vi "Create Robot State Machine.vi"(8 "error in (no error)":errorcluster, 11 "Robot Definition":T1) -> (0 "error out":errorcluster, 3 "Cluster":T2)   [LabVIEW 2014]
uses:
  Robot_creation_loop_data.ctl
  Robot_definition.ctl
  Build robot states.ctl
  <vilib>/picture/3D Picture Control/Object/Create Object (name).vi
  <vilib>/picture/3D Picture Control/Object/Add Object (no reference).vi
  <vilib>/picture/3D Picture Control/Object/Create Object (drawable).vi
  <vilib>/picture/3D Picture Control/Object/Add Object (reference).vi
  <vilib>/picture/3D Picture Control/NI_3D Picture Control.lvlib
panel:
  out "x/y":sgl
  out "Robot Definition.Base":sgl
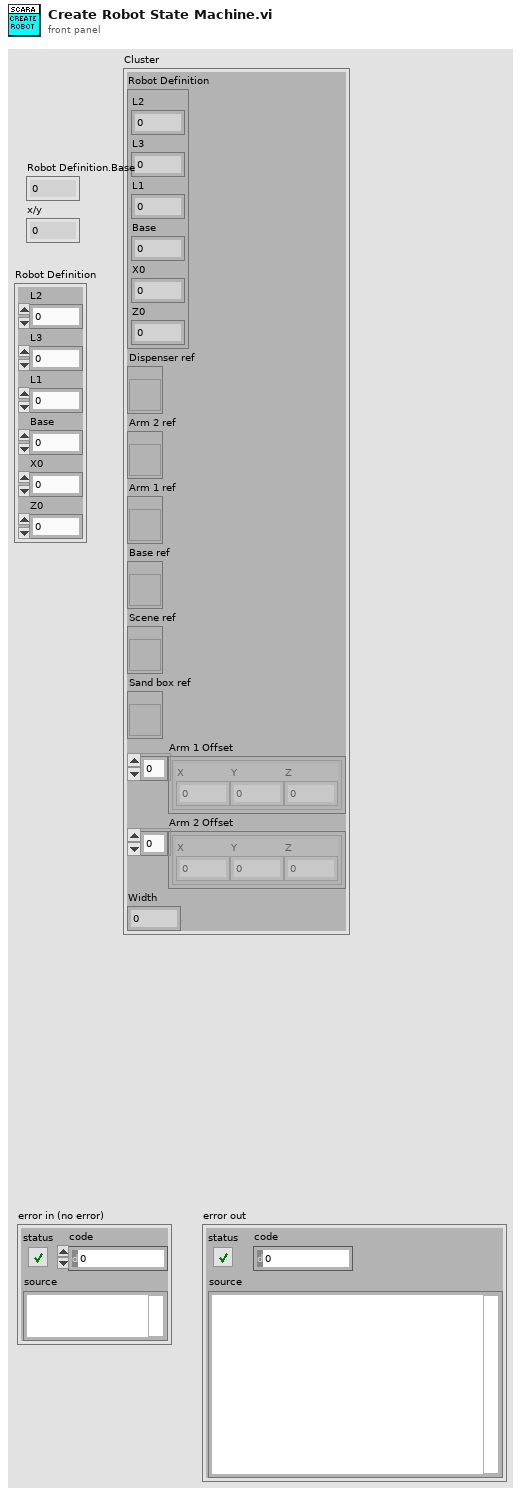
[diagram p1: front panel]
types:
  T1 = typedef "Robot_definition.ctl" = cluster{"L2":sgl, "L3":sgl, "L1":sgl, "Base":sgl, "X0":sgl, "Z0":sgl}
  T2 = typedef "Robot_creation_loop_data.ctl" = cluster{"Robot Definition":T1, "Dispenser ref":refnum<vi>, "Arm 2 ref":refnum<vi>, "Arm 1 ref":refnum<vi>, "Base ref":refnum<vi>, "Scene ref":refnum<vi>, "Sand box ref":refnum<vi>, "Arm 1 Offset":cluster{"X":sgl, "Y":sgl, "Z":sgl}[], "Arm 2 Offset":cluster{"X":sgl, "Y":sgl, "Z":sgl}[], "Width":sgl}
  T3 = typedef "Build robot states.ctl" = enum16{"Init 1 - Clear references", "Create Scene", "Create Sand box", "Create Base", "Create Arm 1", "Create Arm 2", "Create Dispenser", "Exit"}
  T4 = cluster{"Red":sgl, "Green":sgl, "Blue":sgl, "Alpha":sgl}
  T5 = enum16{"Zero", "One", "Destination Color", "One Minus Destination Color", "Source Alpha", "One Minus Source Alpha", "Destination Alpha", "One Minus Destination Alpha", "Source Alpha Saturate"}
  T6 = enum16{"Zero", "One", "Source Color", "One Minus Source Color", "Source Alpha", "One Minus Source Alpha", "Destination Alpha", "One Minus Destination Alpha"}
  T7 = enum16{"Normal Bin", "Opaque Bin", "Transparent Bin"}
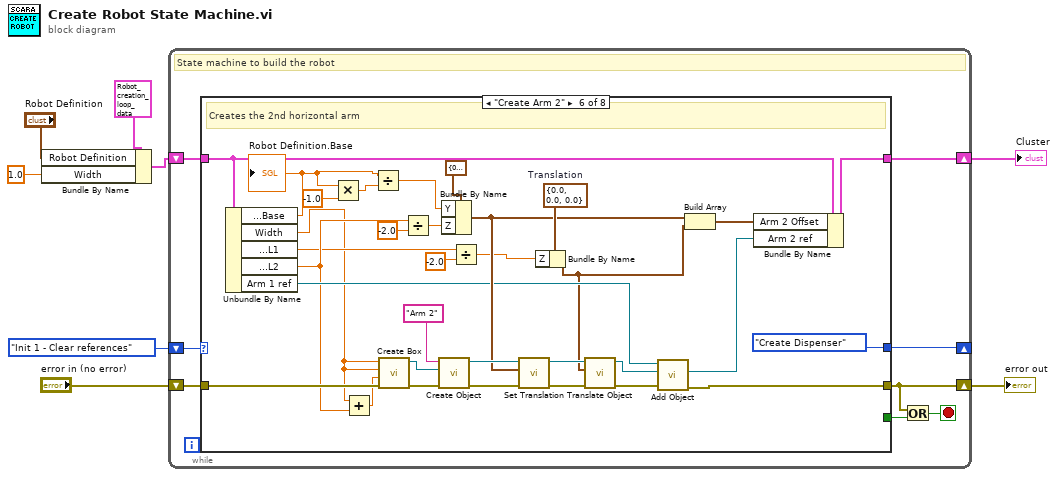
[diagram p0: block diagram]
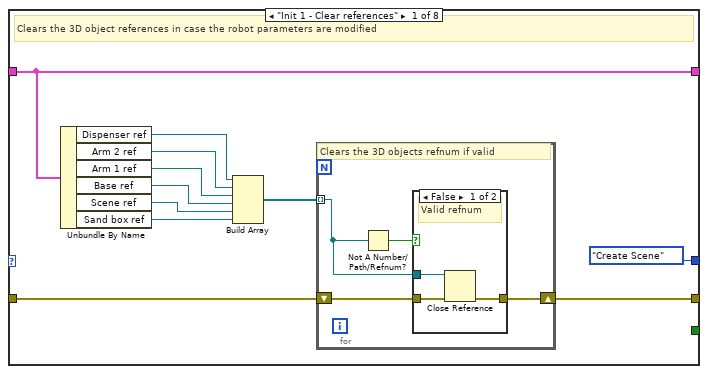
[diagram p2: hidden frame]
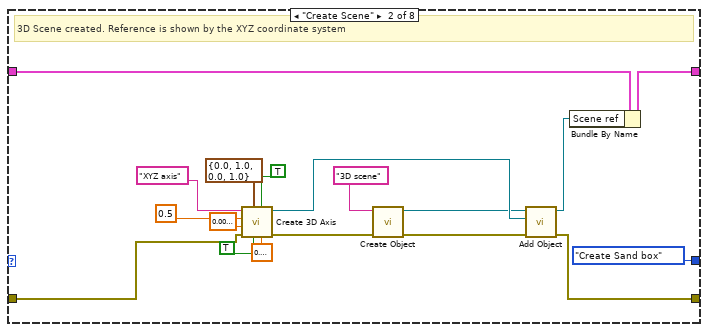
[diagram p4: hidden frame]
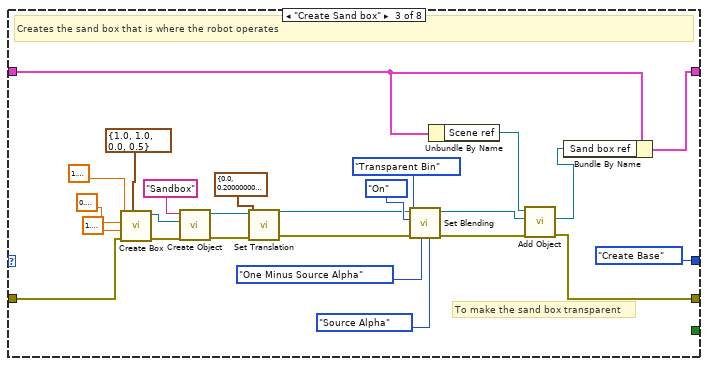
[diagram p5: hidden frame]
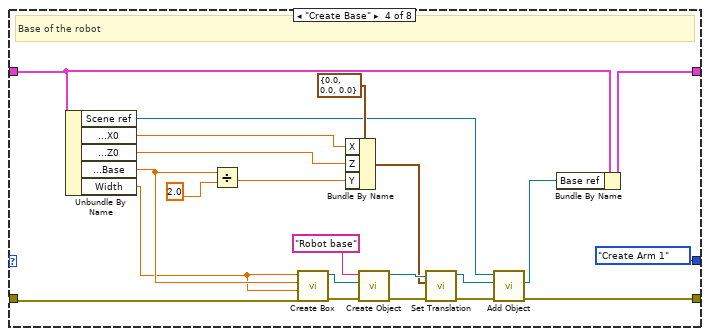
[diagram p6: hidden frame]
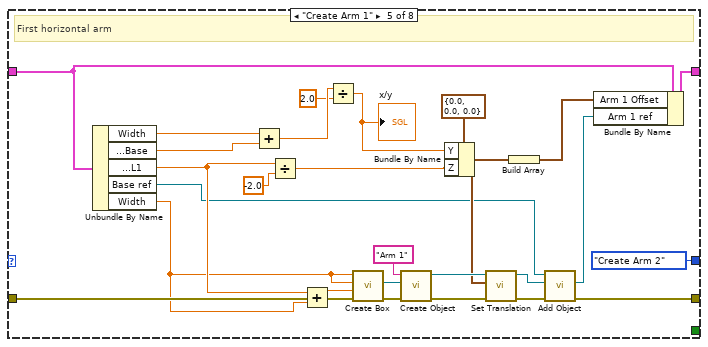
[diagram p7: hidden frame]
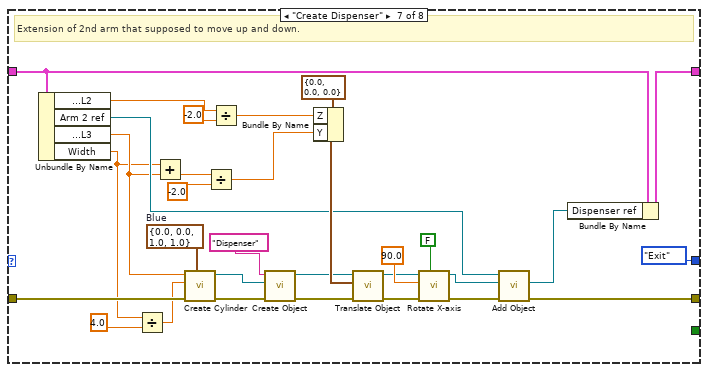
[diagram p8: hidden frame]
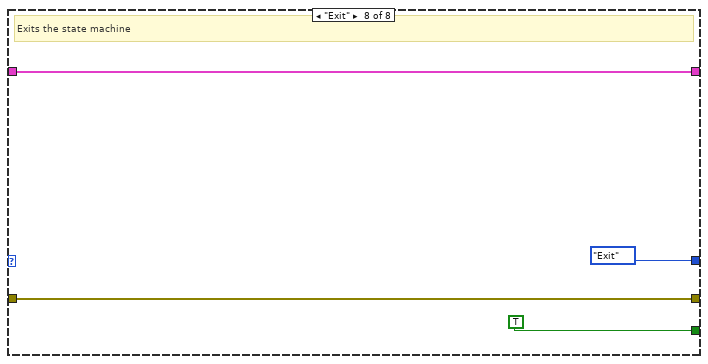
[diagram p9: hidden frame]
diagram:
  n1 = Bundle By Name(cluster=T2 {"Robot Definition"={"L2"=0.0, "L3"=0.0, "L1"=0.0, "Base"=0.0, "X0"=0.0, "Z0"=0.0}, "Dispenser ref"=refnum, "Arm 2 ref"=refnum, "Arm 1 ref"=refnum, "Base ref"=refnum, "Scene ref"=refnum, "Sand box ref"=refnum, "Arm 1 Offset"=[], "Arm 2 Offset"=[], "Width"=0.0}, "Robot Definition"="Robot Definition", "Width"=sgl 1.0) -> (w3:T2)
  n2 = while {
    shift-right: [w9] -> w1
    shift-left: w3 -> [w13]
    shift-right: [w14] -> _
    shift-left: Build_robot_states."Init 1 - Clear references" -> [w16]
    shift-right: [w10] -> w7
    shift-left: "error in (no error)" -> [w12]
    stop <- w11 stop-if-true
    # "State machine to build the robot"
    n3 = case shown="\"Create Arm 2\"" w16 {
      tunnel: [_ _ _ _ _ _ _ TRUE] -> w15
      tunnel: [Build_robot_states."Create Scene" Build_robot_states."Create Sand box" Build_robot_states."Create Base" Build_robot_states."Create Arm 1" Build_robot_states."Create Arm 2" Build_robot_states."Create Dispenser" Build_robot_states."Exit" Build_robot_states."Exit"] -> w14
      tunnel: w13 -> [w27 w41 w61 w88 w119 w152 w176 w193]
      tunnel: [w26 w44 w54 w90 w115 w149 w174 w192] -> w10
      tunnel: w12 -> [w25 w43 w55 w93 w116 w147 w178 w192]
      tunnel: [w27 w40 w57 w87 w112 w150 w175 w193] -> w9
      frame "Init 1 - Clear references" {
        # "Clears the 3D object references in case the robot parameters are modified"
        n4 = Unbundle By Name(w27) -> ("Dispenser ref"=w24:refnum<vi>, "Arm 2 ref"=w23:refnum<vi>, "Arm 1 ref"=w22:refnum<vi>, "Base ref"=w21:refnum<vi>, "Scene ref"=w20:refnum<vi>, "Sand box ref"=w19:refnum<vi>)
        n5 = Build Array(w24, w23, w22, w21, w20, w19) -> (w18:refnum<vi>[])
        n6 = for {
          shift-right: [w30] -> w26
          shift-left: w25 -> [w29]
          tunnel: w18 -> [w28] mode=indexing
          # "Clears the 3D objects refnum if valid"
          n7 = Not A Number/Path/Refnum?(number/path/refnum=w28) -> (NaN/Path/Refnum?=w31:bool)
          n8 = case shown="False" w31 {
            tunnel: [w34 w35] -> w30
            tunnel: w29 -> [w33 w35]
            tunnel: w28 -> [w32 _]
            frame False {
              # "Valid refnum"
              n9 = Close Reference(reference=w32, error in (no error)=w33) -> (error out=w34:errorcluster)
            }
            frame True {
              # "Not a refnum"
            }
          }
        }
      }
      frame "Create Scene" {
        # "3D Scene created. Reference is shown by the XYZ coordinate system"
        n10 = call <vilib>:"Create 3D Axis.vi"("Character Size"=sgl 0.2, "Half plane?"=TRUE, "Axis label?"=TRUE, "Color"=T4 {"Red"=0.0, "Green"=1.0, "Blue"=0.0, "Alpha"=1.0}, "error in (no error)"=w43, "Radius"=sgl 0.01, "Length"=sgl 0.5, "Name"="XYZ axis") -> ("error out"=w36:errorcluster, "New Object Refnum"=w45:refnum<vi>)  [unwired: 2 in]
        n11 = call-poly <vilib>:"Create Object.vi"("error in (no error)"=w36, "Name"="3D scene") -> ("error out"=w37:errorcluster, "Scene:New Object"=w38:refnum<vi>)  [unwired: 8 in]
        n12 = call-poly <vilib>:"Add Object.vi"("error in (no error)"=w37, "New Object In"=w45, "Scene Object In"=w38) -> ("error out"=w44:errorcluster, "Scene Object Out"=w39:refnum<vi>)  [unwired: 7 in]
        n13 = Bundle By Name(cluster=w41, "Scene ref"=w39) -> (w40:T2)
      }
      frame "Create Sand box" {
        # "To make the sand box transparent"
        # "Creates the sand box that is where the robot operates"
        n14 = call <vilib>:"Create Box.vi"("Color"=T4 {"Red"=1.0, "Green"=1.0, "Blue"=0.0, "Alpha"=0.5}, "error in (no error)"=w55, "Length Z"=sgl 1.3, "Length Y"=sgl 0.4, "Length X"=sgl 1.8) -> ("error out"=w66:errorcluster, "New Box Refnum"=w69:refnum<vi>)  [unwired: 5 in]
        n15 = call-poly <vilib>:"Create Object.vi"("error in (no error)"=w66, "Geometry"=w69, "Name"="Sandbox") -> ("error out"=w65:errorcluster, "Scene:New Object"=w64:refnum<vi>)  [unwired: 7 in]
        n16 = call <vilib>:"Set Translation.vi"("error in (no error)"=w65, "Translation"=cluster{"X":sgl, "Y":sgl, "Z":sgl} {"X"=0.0, "Y"=0.2, "Z"=0.0}, "Scene Object"=w64) -> ("error out"=w73:errorcluster, "Translated Object"=w72:refnum<vi>)  [unwired: 7 in]
        n17 = call <vilib>:"Set Blending.vi"("Source"=T5."Source Alpha", "Destination"=T6."One Minus Source Alpha", "error in (no error)"=w73, "Bin"=T7."Transparent Bin", "Mode"=enum16{"Inherit Value", "Off", "On"}."On", "Scene Object In"=w72) -> ("error out"=w62:errorcluster, "Scene Object Out"=w59:refnum<vi>)  [unwired: 4 in]
        n18 = Unbundle By Name(w61) -> ("Scene ref"=w60:refnum<vi>)
        n19 = call-poly <vilib>:"Add Object.vi"("error in (no error)"=w62, "New Object In"=w59, "Scene Object In"=w60) -> ("error out"=w54:errorcluster, "New Object Out"=w58:refnum<vi>)  [unwired: 6 in, 1 out]
        n20 = Bundle By Name(cluster=w61, "Sand box ref"=w58) -> (w57:T2)
      }
      frame "Create Base" {
        # "Base of the robot"
        n21 = Unbundle By Name(w88) -> ("Scene ref"=w83:refnum<vi>, "Robot Definition.X0"=w80:sgl, "Robot Definition.Z0"=w79:sgl, "Robot Definition.Base"=w95:sgl, "Width"=w81:sgl)
        n22 = Divide(x=w95, y=sgl 2.0 ("x")) -> (x/y=w85:sgl)
        n23 = call <vilib>:"Create Box.vi"("error in (no error)"=w93, "Length Z"=w81, "Length Y"=w95, "Length X"=w81) -> ("error out"=w97:errorcluster, "New Box Refnum"=w96:refnum<vi>)  [unwired: 6 in]
        n24 = Bundle By Name(cluster=cluster{"X":sgl, "Y":sgl, "Z":sgl} {"X"=0.0, "Y"=0.0, "Z"=0.0} ("Translation"), "X"=w80, "Z"=w79, "Y"=w85) -> (w94:cluster{"X":sgl, "Y":sgl, "Z":sgl})
        n25 = call-poly <vilib>:"Create Object.vi"("error in (no error)"=w97, "Geometry"=w96, "Name"="Robot base") -> ("error out"=w98:errorcluster, "Scene:New Object"=w99:refnum<vi>)  [unwired: 7 in]
        n26 = call <vilib>:"Set Translation.vi"("error in (no error)"=w98, "Translation"=w94, "Scene Object"=w99) -> ("error out"=w100:errorcluster, "Translated Object"=w82:refnum<vi>)  [unwired: 7 in]
        n27 = call-poly <vilib>:"Add Object.vi"("error in (no error)"=w100, "New Object In"=w82, "Scene Object In"=w83) -> ("error out"=w90:errorcluster, "New Object Out"=w84:refnum<vi>)  [unwired: 6 in, 1 out]
        n28 = Bundle By Name(cluster=w88, "Base ref"=w84) -> (w87:T2)
      }
      frame "Create Arm 1" {
        # "First horizontal arm"
        n29 = Unbundle By Name(w119) -> ("Width"=w104:sgl, "Robot Definition.Base"=w105:sgl, "Robot Definition.L1"=w114:sgl, "Base ref"=w108:refnum<vi>, "Width"=w106:sgl)
        n30 = Add(x=w104, y=w105) -> (x+y=w103:sgl)
        n31 = Divide(x=w114, y=sgl -2.0) -> (x/y=w113:sgl)
        n32 = Add(x=w114, y=w106) -> (x+y=w127:sgl)
        n33 = Divide(x=w103, y=sgl 2.0) -> (x/y=w102:sgl)
        "x/y" <- w102
        n34 = call <vilib>:"Create Box.vi"("error in (no error)"=w116, "Length Z"=w127, "Length Y"=w106, "Length X"=w106) -> ("error out"=w122:errorcluster, "New Box Refnum"=w121:refnum<vi>)  [unwired: 6 in]
        n35 = call-poly <vilib>:"Create Object.vi"("error in (no error)"=w122, "Geometry"=w121, "Name"="Arm 1") -> ("error out"=w123:errorcluster, "Scene:New Object"=w125:refnum<vi>)  [unwired: 7 in]
        n36 = Bundle By Name(cluster=cluster{"X":sgl, "Y":sgl, "Z":sgl} {"X"=0.0, "Y"=0.0, "Z"=0.0} ("Translation"), "Y"=w102, "Z"=w113) -> (w117:cluster{"X":sgl, "Y":sgl, "Z":sgl})
        n37 = call <vilib>:"Set Translation.vi"("error in (no error)"=w123, "Translation"=w117, "Scene Object"=w125) -> ("error out"=w124:errorcluster, "Translated Object"=w107:refnum<vi>)  [unwired: 7 in]
        n38 = Build Array(w117) -> (w111:cluster{"X":sgl, "Y":sgl, "Z":sgl}[])
        n39 = call-poly <vilib>:"Add Object.vi"("error in (no error)"=w124, "New Object In"=w107, "Scene Object In"=w108) -> ("error out"=w115:errorcluster, "New Object Out"=w109:refnum<vi>)  [unwired: 6 in, 1 out]
        n40 = Bundle By Name(cluster=w119, "Arm 1 Offset"=w111, "Arm 1 ref"=w109) -> (w112:T2)
      }
      frame "Create Arm 2" {
        w160 = cluster{"X":sgl, "Y":sgl, "Z":sgl} {"X"=0.0, "Y"=0.0, "Z"=0.0}  # Translation
        # "Creates the 2nd horizontal arm"
        n41 = Unbundle By Name(w152) -> ("Robot Definition.Base"=w129:sgl, "Width"=w132:sgl, "Robot Definition.L1"=w135:sgl, "Robot Definition.L2"=w138:sgl, "Arm 1 ref"=w145:refnum<vi>)
        "Robot Definition.Base" <- w129
        n42 = Multiply(x=w129, y=sgl -1.0) -> (x*y=w130:sgl)
        n43 = Add(x=w132, y=w138) -> (x+y=w140:sgl)
        n44 = Divide(x=w129, y=w130) -> (x/y=w131:sgl)
        n45 = call <vilib>:"Create Box.vi"("error in (no error)"=w147, "Length Z"=w140, "Length Y"=w132, "Length X"=w132) -> ("error out"=w154:errorcluster, "New Box Refnum"=w157:refnum<vi>)  [unwired: 6 in]
        n46 = Divide(x=w138, y=sgl -2.0 ("x")) -> (x/y=w134:sgl)
        n47 = call-poly <vilib>:"Create Object.vi"("error in (no error)"=w154, "Geometry"=w157, "Name"="Arm 2") -> ("error out"=w155:errorcluster, "Scene:New Object"=w156:refnum<vi>)  [unwired: 7 in]
        n48 = Bundle By Name(cluster=cluster{"X":sgl, "Y":sgl, "Z":sgl} {"X"=0.0, "Y"=0.0, "Z"=0.0} ("Translation"), "Y"=w131, "Z"=w134) -> (w151:cluster{"X":sgl, "Y":sgl, "Z":sgl})
        n49 = Divide(x=w135, y=sgl -2.0 ("x")) -> (x/y=w133:sgl)
        n50 = call <vilib>:"Set Translation.vi"("error in (no error)"=w155, "Translation"=w151, "Scene Object"=w156) -> ("error out"=w141:errorcluster, "Translated Object"=w142:refnum<vi>)  [unwired: 7 in]
        n51 = Bundle By Name(cluster=w160, "Z"=w133) -> (w139:cluster{"X":sgl, "Y":sgl, "Z":sgl})
        n52 = call <vilib>:"Translate Object.vi"("error in (no error)"=w141, "Translation"=w139, "Scene.Object In"=w142) -> ("error out"=w159:errorcluster, "Scene.Object Out"=w144:refnum<vi>)  [unwired: 7 in]
        n53 = call-poly <vilib>:"Add Object.vi"("error in (no error)"=w159, "New Object In"=w144, "Scene Object In"=w145) -> ("error out"=w149:errorcluster, "New Object Out"=w143:refnum<vi>)  [unwired: 6 in, 1 out]
        n54 = Build Array(w151, w139) -> (w146:cluster{"X":sgl, "Y":sgl, "Z":sgl}[])
        n55 = Bundle By Name(cluster=w152, "Arm 2 Offset"=w146, "Arm 2 ref"=w143) -> (w150:T2)
      }
      frame "Create Dispenser" {
        w190 = T4 {"Red"=0.0, "Green"=0.0, "Blue"=1.0, "Alpha"=1.0}  # Blue
        # "Extension of 2nd arm that supposed to move up and down."
        n56 = Unbundle By Name(w176) -> ("Robot Definition.L2"=w170:sgl, "Arm 2 ref"=w171:refnum<vi>, "Robot Definition.L3"=w166:sgl, "Width"=w163:sgl)
        n57 = Divide(x=w163, y=sgl 4.0 ("x")) -> (x/y=w162:sgl)
        n58 = Add(x=w163, y=w166) -> (x+y=w164:sgl)
        n59 = call <vilib>:"Create Cylinder.vi"("Color"=w190, "error in (no error)"=w178, "Radius"=w162, "Height"=w166) -> ("error out"=w181:errorcluster, "New Cylinder Refnum"=w183:refnum<vi>)  [unwired: 6 in]
        n60 = Divide(x=w164, y=sgl -2.0 ("x")) -> (x/y=w167:sgl)
        n61 = Divide(x=w170, y=sgl -2.0 ("x")) -> (x/y=w169:sgl)
        n62 = call-poly <vilib>:"Create Object.vi"("error in (no error)"=w181, "Geometry"=w183, "Name"="Dispenser") -> ("error out"=w184:errorcluster, "Scene:New Object"=w182:refnum<vi>)  [unwired: 7 in]
        n63 = Bundle By Name(cluster=cluster{"X":sgl, "Y":sgl, "Z":sgl} {"X"=0.0, "Y"=0.0, "Z"=0.0} ("Translation"), "Z"=w169, "Y"=w167) -> (w191:cluster{"X":sgl, "Y":sgl, "Z":sgl})
        n64 = call <vilib>:"Translate Object.vi"("error in (no error)"=w184, "Translation"=w191, "Scene.Object In"=w182) -> ("error out"=w186:errorcluster, "Scene.Object Out"=w187:refnum<vi>)  [unwired: 7 in]
        n65 = call <vilib>:"Rotate X-axis.vi"("Relative?"=FALSE, "error in (no error)"=w186, "angle"=90.0, "Scene Object In"=w187) -> ("error out"=w179:errorcluster, "Scene Object Out"=w173:refnum<vi>)  [unwired: 6 in]
        n66 = call-poly <vilib>:"Add Object.vi"("error in (no error)"=w179, "New Object In"=w173, "Scene Object In"=w171) -> ("error out"=w174:errorcluster, "New Object Out"=w172:refnum<vi>)  [unwired: 6 in, 1 out]
        n67 = Bundle By Name(cluster=w176, "Dispenser ref"=w172) -> (w175:T2)
      }
      frame "Exit" {
        # "Exits the state machine"
      }
    }
    n68 = Or(x=w10, y=w15) -> (x .or. y?=w11:bool)
  }
  "Cluster" <- w1
  "error out" <- w7
